vi "Untitled 2.vi"() -> ()   [LabVIEW 2015]
panel:
  in  "PID Gains":T1={"proportional gain (Kc)"=1.3979250340642948, "integral time (Ti, min)"=2.9580260274160532, "derivative time (Td, min)"=0.46155392250462524} {"derivative time (Td, min)" format="%#.6g"; "integral time (Ti, min)" format="%#.6g"; "proportional gain (Kc)" format="%#.6g"}
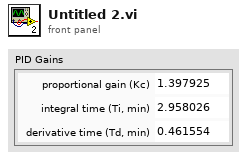
[diagram p1: front panel]
types:
  T1 = cluster{"proportional gain (Kc)":dbl, "integral time (Ti, min)":dbl, "derivative time (Td, min)":dbl}
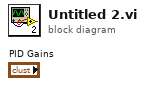
[diagram p0: block diagram]
diagram:
